vi "Read Index.vi"(8 "error in (no error)":errorcluster, 11 "Local Bus_DBL in":refnum<class "Local Bus_U64.lvclass">) -> (0 "error out":errorcluster, 2 "Index":i32, 3 "Local Bus_DBL out":refnum<class "Local Bus_U64.lvclass">)   [LabVIEW 2021, in "Local Bus_U64.lvclass"]
uses:
  Local Bus_U64.lvclass
  Local Bus_U64.lvclass/Local Bus_U64.ctl
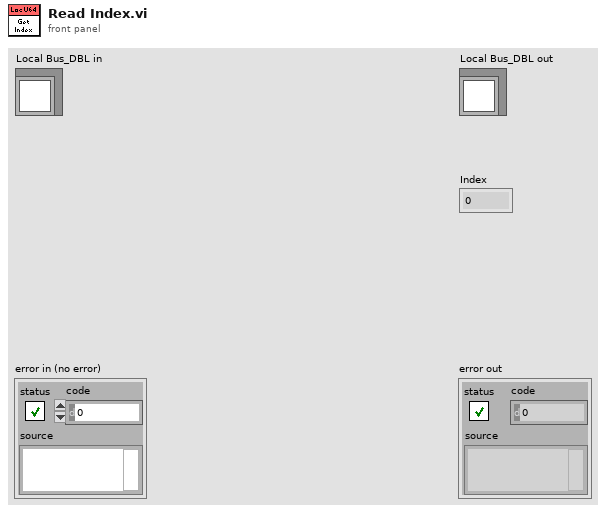
[diagram p1: front panel]
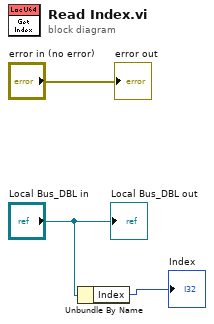
[diagram p0: block diagram]
diagram:
  n1 = Unbundle By Name("Local Bus_DBL in") -> ("Index"=→"Index":i32)
  "error out" <- "error in (no error)"
  "Local Bus_DBL out" <- "Local Bus_DBL in"
